vi "replaceQueryTokens.vi"(8 "error in (no error)":errorcluster, 10 "Querry In":string, 11 "Goal in":refnum<class "Goal.lvclass">) -> (0 "error out":errorcluster, 2 "Query Out":string, 3 "Goal out":refnum<class "Goal.lvclass">)   [LabVIEW 2020, in "Goal.lvclass"]
uses:
  Goal.lvclass
  Goal.lvclass/Goal.ctl
  WhichMonth/WhichMonth.lvclass
  Category/Category.lvclass
  UserEditableAmount/UserEditableAmount.lvclass
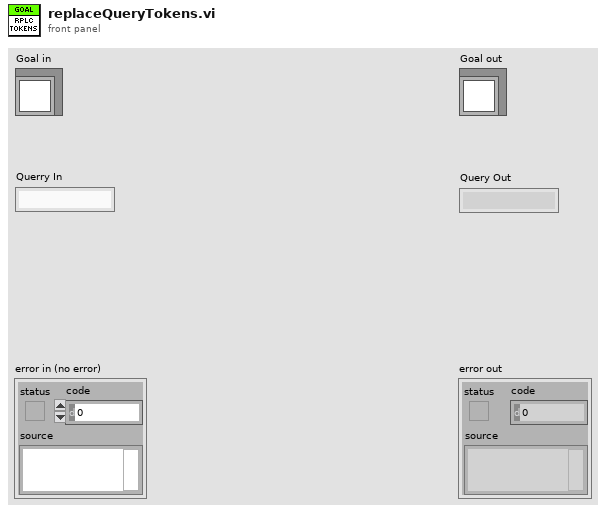
[diagram p1: front panel]
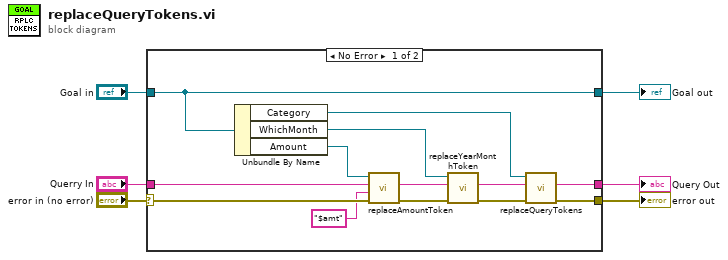
[diagram p0: block diagram]
diagram:
  n1 = case shown="No Error" "error in (no error)" {
    selector: "error in (no error)" -> [w10 w22]
    tunnel: [w13 w22] -> w5
    tunnel: [w15 w21] -> w3
    tunnel: "Goal in" -> [w15 w21]
    tunnel: [w14 w20] -> w2
    tunnel: "Querry In" -> [w9 w20]
    frame No Error {
      n2 = Unbundle By Name(w15) -> ("Category"=w18:refnum<class "Category.lvclass">, "WhichMonth"=w19:refnum<class "WhichMonth.lvclass">, "Amount"=w12:refnum<class "UserEditableAmount.lvclass">)
      n3 = call "replaceAmountToken.vi"("error in (no error)"=w10, "amt token"="$amt" ("search string"), "Query In"=w9, "UserEditableAmount in"=w12) -> ("error out"=w11:errorcluster, "Query Out"=w8:string)  [unwired: 5 in, 1 out]
      n4 = call "replaceYearMonthToken.vi"("error in (no error)"=w11, "Query In"=w8, "WhichMonth in"=w19) -> ("error out"=w16:errorcluster, "Query Out"=w17:string)  [unwired: 6 in, 1 out]
      n5 = call "replaceQueryTokens.vi"("error in (no error)"=w16, "Query In"=w17, "Category in"=w18) -> ("error out"=w13:errorcluster, "Query Out"=w14:string)  [unwired: 6 in, 1 out]
    }
    frame Error {
    }
  }
  "error out" <- w5
  "Goal out" <- w3
  "Query Out" <- w2
